vi "RelayBoard_16in16out_ZQ_TestStand.vi"(8 "On/Off":bool, 9 "Index":dbl, 10 "功能":T1(ring), 11 "ComPort":string) -> (2 "DI Status":bool, 3 "数组":bool[](array[boolean]))   [LabVIEW 2018]
uses:
  <vilib>/Instr/_visa.llb/VISA Configure Serial Port (Instr).vi
panel:
  out "数组 2":bool[](array[boolean])
  out "连接状态":bool
  in  "全部断开":bool
  in  "全部闭合":bool
  in  "OUT 16":bool
  in  "OUT 15":bool
  in  "OUT 14":bool
  in  "OUT 13":bool
  in  "OUT 12":bool
  in  "OUT 11":bool
  in  "OUT 10":bool
  in  "OUT 9":bool
  in  "OUT 8":bool
  in  "OUT 7":bool
  in  "OUT 6":bool
  in  "OUT 5":bool
  in  "OUT 4":bool
  in  "OUT 3":bool
  in  "打开端口":bool
  in  "停止":bool
  in  "OUT 2":bool
  in  "OUT 1":bool
  in  "VISA resource name":refnum<visa-resource-name> caption="VISA资源名称"
  # "智嵌IO控制板_调用"
  # "X1"
  # "X2"
  # "X3"
  # "X4"
  # "X5"
  # "X6"
  # "X7"
  # "X8"
  # "X9"
  # "X10"
  # "X11"
  # "X12"
  # "X13"
  # "X14"
  # "X15"
  # "X16"
  # "X1"
  # "X2"
  # "X3"
  # "X4"
  # "X5"
  # "X6"
  # "X7"
  # "X8"
  # "X9"
  # "X10"
  # "X11"
  # "X12"
  # "X13"
  # "X14"
  # "X15"
  # "X16"
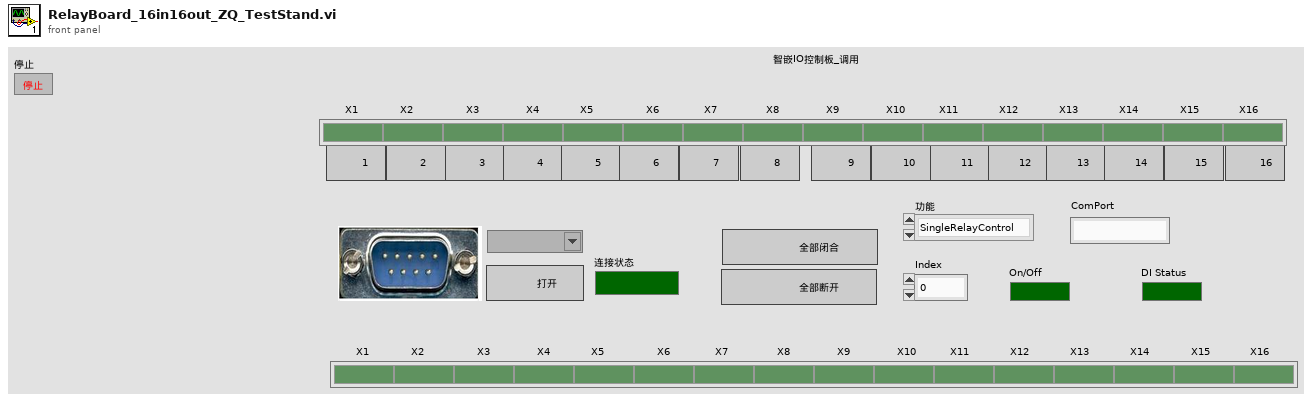
[diagram p1: front panel]
types:
  T1 = enum16{"SingleRelayControl", "AllRelaysControl", "OpenComPort", "CloseComPort", "ReadDI"}
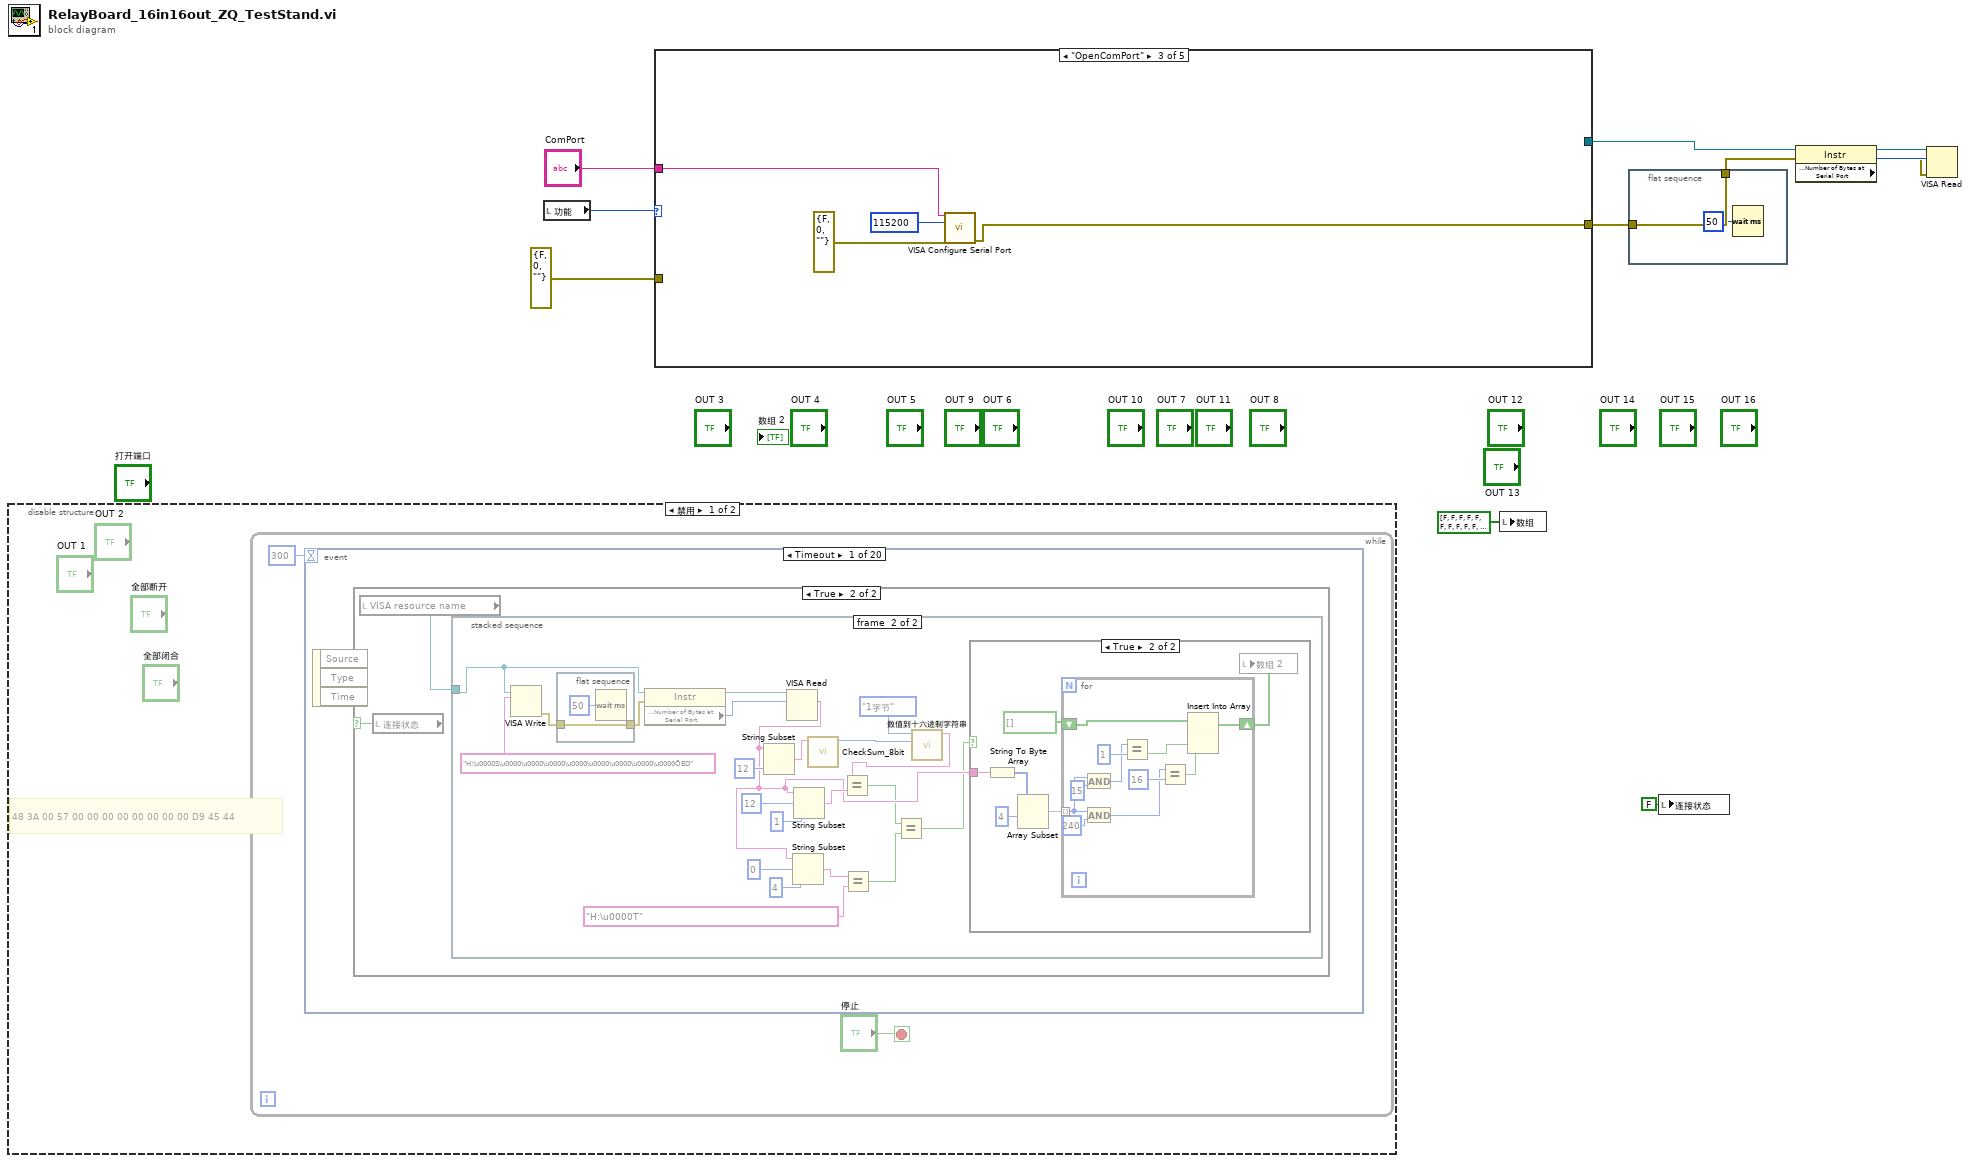
[diagram p0: block diagram]
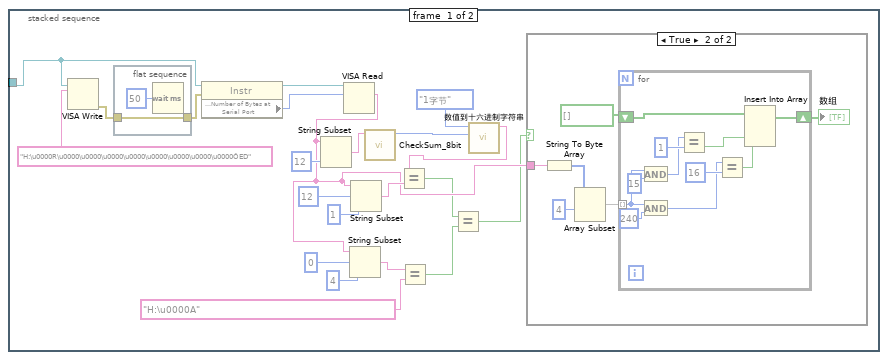
[diagram p3: hidden frame]
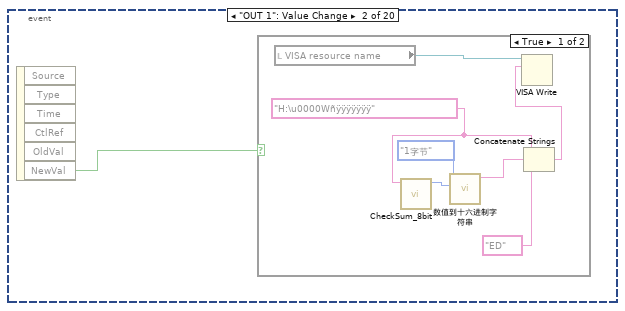
[diagram p6: hidden frame]
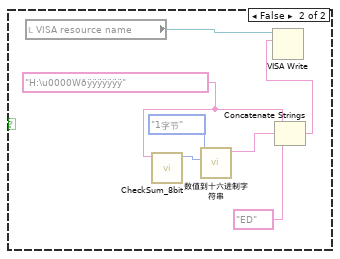
[diagram p7: hidden frame]
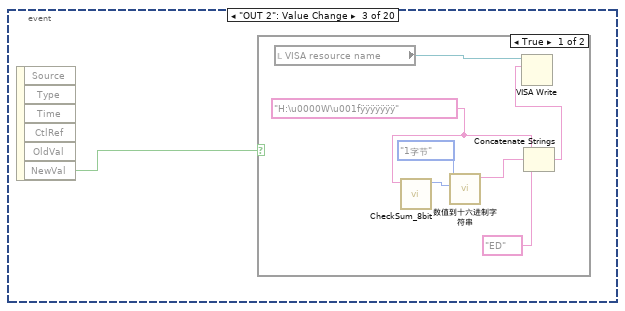
[diagram p8: hidden frame]
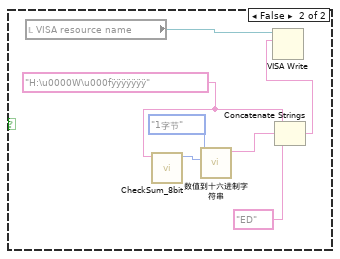
[diagram p9: hidden frame]
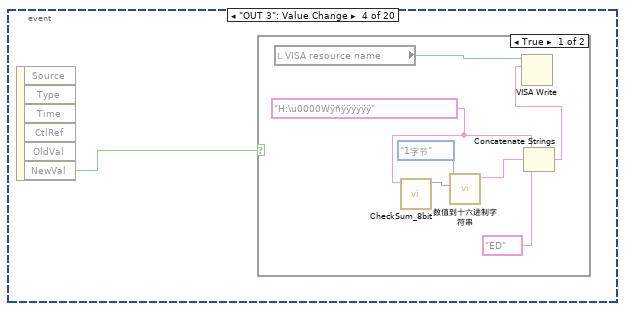
[diagram p10: hidden frame]
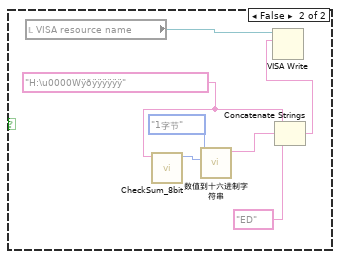
[diagram p11: hidden frame]
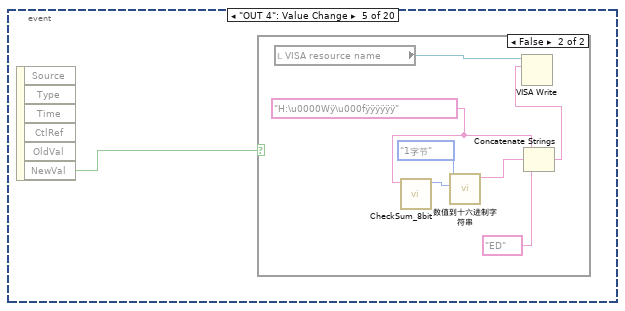
[diagram p12: hidden frame]
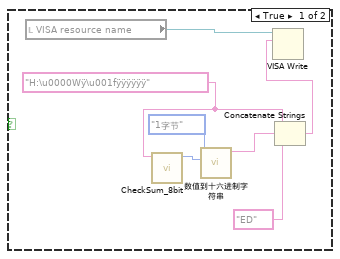
[diagram p13: hidden frame]
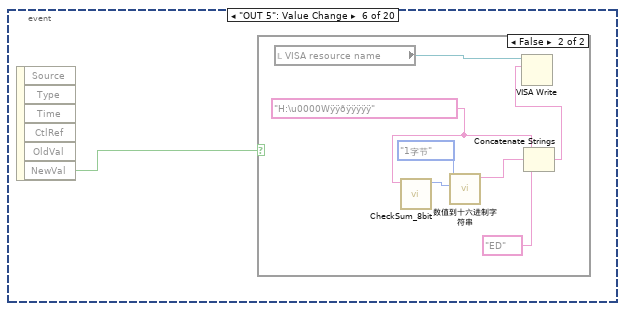
[diagram p14: hidden frame]
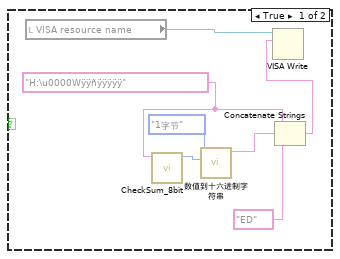
[diagram p15: hidden frame]
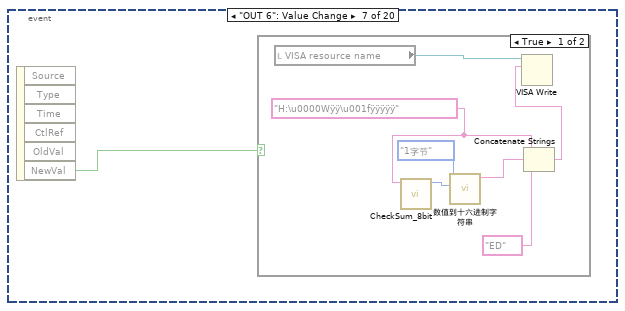
[diagram p16: hidden frame]
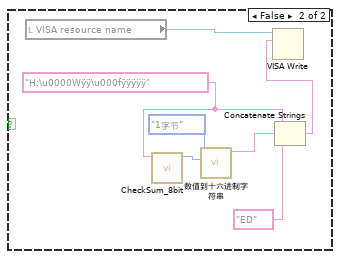
[diagram p17: hidden frame]
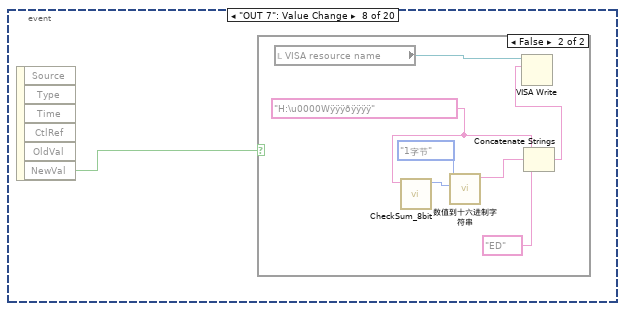
[diagram p18: hidden frame]
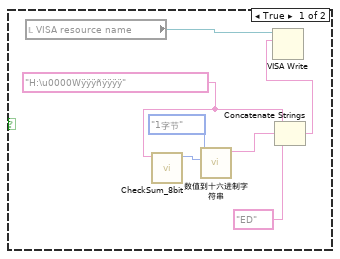
[diagram p19: hidden frame]
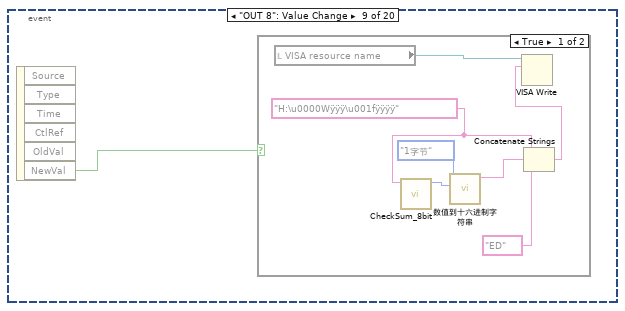
[diagram p20: hidden frame]
diagram:
  n1 = disable-structure shown="禁用" {
    frame Disabled {
      # "48 3A 00 57 00 00 00 00 00 00 00 00 D9 45 44"
      n2 = while {
        stop <- "停止" stop-if-true
        n3 = event shown="[0] Timeout" {
          selector: _ -> [_ _ _ _ _ _ _ _ _ _ _ _ _ _ _ _ _ _ _ _]
          dyn-events: _ -> [_ _ _ _ _ _ _ _ _ _ _ _ _ _ _ _ _ _ _ _]
          timeout: 300 -> [_ _ _ _ _ _ _ _ _ _ _ _ _ _ _ _ _ _ _ _]
          event Timeout {
            n4 = event-data() -> ()  [unwired: 1 in, 3 out]
            n5 = local read "连接状态"() -> (w14:bool)
            n6 = case shown="True" w14 {
              frame False {
              }
              frame True {
                n7 = local read "VISA resource name"() -> (w15:refnum<visa-resource-name>)
                n8 = stacked-sequence {
                  tunnel: w15 -> [w32 w73]
                  frame #0 {
                    n9 = VISA Write(VISA resource name=w32, write buffer="H:\u0000R\u0000\u0000\u0000\u0000\u0000\u0000\u0000\u0000ÔED" ("写入缓冲区")) -> (error out=w33:errorcluster)  [unwired: 1 in, 2 out]
                    n10 = flat-sequence {
                      tunnel: [w38] -> w34
                      tunnel: w33 -> [w38]
                      frame #0 {
                        n11 = Wait (ms)(milliseconds to wait=u32 50 ("等待时间（毫秒）")) -> ()  [unwired: 1 out]
                      }
                    }
                    n12 = property class="Instr"(reference=w32, error in=w34) -> (reference out=w37:refnum<visa-resource-name>, "Serial Settings:Number of Bytes at Serial Port"=w36:u32)  [unwired: 1 out]
                    n13 = VISA Read(VISA resource name=w37, byte count=w36) -> (read buffer=w21:string)  [unwired: 1 in, 3 out]
                    n14 = String Subset(string=w21, length (rest)=12 ("长度（剩余）")) -> (substring=w27:string)  [unwired: 1 in]
                    n15 = String Subset(string=w21, offset (0)=0 ("偏移量(0)"), length (rest)=4 ("长度（剩余）")) -> (substring=w20:string)
                    n16 = String Subset(string=w21, offset (0)=12 ("偏移量(0)"), length (rest)=1 ("长度（剩余）")) -> (substring=w28:string)
                    n17 = call "CheckSum_8bit.vi"("字符串"=w27) -> ("和"=w25:u32)  [unwired: 10 in]
                    n18 = Equal?(x=w20, y="H:\u0000A" ("写入缓冲区")) -> (x = y?=w17:bool)
                    n19 = call "数值到十六进制字符串.vi"("Numeric"=w25, "转换字节数"=enum16{"1字节", "2字节", "4字节", "3字节"}."1字节") -> ("转换结果"=w24:string)  [unwired: 8 in, 1 out]
                    n20 = Equal?(x=w24, y=w28) -> (x = y?=w18:bool)
                    n21 = Equal?(x=w18, y=w17) -> (x = y?=w16:bool)
                    n22 = case shown="True" w16 {
                      tunnel: w21 -> [_ w45]
                      frame False {
                      }
                      frame True {
                        n23 = String To Byte Array(string=w45) -> (unsigned byte array=w44:u8[])
                        n24 = Array Subset(array=w44, index=4 ("索引")) -> (w42:u8[])  [unwired: 1 in]
                        n25 = for {
                          tunnel: w42 -> [w49] mode=indexing
                          shift-right: [w51] -> w40
                          shift-left: bool[] [] -> [w54]
                          n26 = And(x=w49, y=u8 15) -> (x .and. y?=w47:u8)
                          n27 = And(x=w49, y=u8 240) -> (x .and. y?=w46:u8)
                          n28 = Equal?(x=w47, y=u8 1) -> (x = y?=w53:bool)
                          n29 = Equal?(x=w46, y=u8 16) -> (x = y?=w52:bool)
                          n30 = Insert Into Array(array=w54, new element #1=w53, new element #2=w52) -> (w51:bool[])  [unwired: 1 in]
                        }
                        "数组" <- w40
                      }
                    }
                  }
                  frame #1 {
                    n31 = VISA Write(VISA resource name=w73, write buffer="H:\u0000S\u0000\u0000\u0000\u0000\u0000\u0000\u0000\u0000ÕED" ("写入缓冲区")) -> (error out=w74:errorcluster)  [unwired: 1 in, 2 out]
                    n32 = flat-sequence {
                      tunnel: [w79] -> w75
                      tunnel: w74 -> [w79]
                      frame #0 {
                        n33 = Wait (ms)(milliseconds to wait=u32 50 ("等待时间（毫秒）")) -> ()  [unwired: 1 out]
                      }
                    }
                    n34 = property class="Instr"(reference=w73, error in=w75) -> (reference out=w78:refnum<visa-resource-name>, "Serial Settings:Number of Bytes at Serial Port"=w77:u32)  [unwired: 1 out]
                    n35 = VISA Read(VISA resource name=w78, byte count=w77) -> (read buffer=w62:string)  [unwired: 1 in, 3 out]
                    n36 = String Subset(string=w62, length (rest)=12 ("长度（剩余）")) -> (substring=w68:string)  [unwired: 1 in]
                    n37 = String Subset(string=w62, offset (0)=0 ("偏移量(0)"), length (rest)=4 ("长度（剩余）")) -> (substring=w61:string)
                    n38 = String Subset(string=w62, offset (0)=12 ("偏移量(0)"), length (rest)=1 ("长度（剩余）")) -> (substring=w69:string)
                    n39 = call "CheckSum_8bit.vi"("字符串"=w68) -> ("和"=w66:u32)  [unwired: 10 in]
                    n40 = Equal?(x=w61, y="H:\u0000T" ("写入缓冲区")) -> (x = y?=w58:bool)
                    n41 = call "数值到十六进制字符串.vi"("Numeric"=w66, "转换字节数"=enum16{"1字节", "2字节", "4字节", "3字节"}."1字节") -> ("转换结果"=w65:string)  [unwired: 8 in, 1 out]
                    n42 = Equal?(x=w65, y=w69) -> (x = y?=w59:bool)
                    n43 = Equal?(x=w59, y=w58) -> (x = y?=w57:bool)
                    n44 = case shown="True" w57 {
                      tunnel: w62 -> [_ w86]
                      frame False {
                      }
                      frame True {
                        n45 = String To Byte Array(string=w86) -> (unsigned byte array=w85:u8[])
                        n46 = Array Subset(array=w85, index=4 ("索引")) -> (w83:u8[])  [unwired: 1 in]
                        n47 = for {
                          tunnel: w83 -> [w90] mode=indexing
                          shift-right: [w92] -> w81
                          shift-left: bool[] [] -> [w95]
                          n48 = And(x=w90, y=u8 15) -> (x .and. y?=w88:u8)
                          n49 = And(x=w90, y=u8 240) -> (x .and. y?=w87:u8)
                          n50 = Equal?(x=w88, y=u8 1) -> (x = y?=w94:bool)
                          n51 = Equal?(x=w87, y=u8 16) -> (x = y?=w93:bool)
                          n52 = Insert Into Array(array=w95, new element #1=w94, new element #2=w93) -> (w92:bool[])  [unwired: 1 in]
                        }
                        n53 = local write "数组 2"(w81) -> ()
                      }
                    }
                  }
                }
              }
            }
          }
          event "OUT 1": Value Change {
            n54 = event-data() -> ("NewVal"=w98:bool)  [unwired: 1 in, 5 out]
            n55 = case shown="True" w98 {
              frame True {
                w99 = "H:\u0000Wñÿÿÿÿÿÿÿ" ("写入缓冲区")
                n56 = local read "VISA resource name"() -> (w105:refnum<visa-resource-name>)
                n57 = call "CheckSum_8bit.vi"("字符串"=w99) -> ("和"=w104:u32)  [unwired: 10 in]
                n58 = call "数值到十六进制字符串.vi"("Numeric"=w104, "转换字节数"=enum16{"1字节", "2字节", "4字节", "3字节"}."1字节") -> ("转换结果"=w102:string)  [unwired: 8 in, 1 out]
                n59 = Concatenate Strings(w99, w102, "ED" ("写入缓冲区")) -> (w100:string)
                n60 = VISA Write(VISA resource name=w105, write buffer=w100) -> ()  [unwired: 1 in, 3 out]
              }
              frame False {
                w106 = "H:\u0000Wðÿÿÿÿÿÿÿ" ("写入缓冲区")
                n61 = local read "VISA resource name"() -> (w112:refnum<visa-resource-name>)
                n62 = call "CheckSum_8bit.vi"("字符串"=w106) -> ("和"=w111:u32)  [unwired: 10 in]
                n63 = call "数值到十六进制字符串.vi"("Numeric"=w111, "转换字节数"=enum16{"1字节", "2字节", "4字节", "3字节"}."1字节") -> ("转换结果"=w109:string)  [unwired: 8 in, 1 out]
                n64 = Concatenate Strings(w106, w109, "ED" ("写入缓冲区")) -> (w107:string)
                n65 = VISA Write(VISA resource name=w112, write buffer=w107) -> ()  [unwired: 1 in, 3 out]
              }
            }
          }
          event "OUT 2": Value Change {
            n66 = event-data() -> ("NewVal"=w113:bool)  [unwired: 1 in, 5 out]
            n67 = case shown="True" w113 {
              frame True {
                w114 = "H:\u0000W\u001fÿÿÿÿÿÿÿ" ("写入缓冲区")
                n68 = local read "VISA resource name"() -> (w120:refnum<visa-resource-name>)
                n69 = call "CheckSum_8bit.vi"("字符串"=w114) -> ("和"=w119:u32)  [unwired: 10 in]
                n70 = call "数值到十六进制字符串.vi"("Numeric"=w119, "转换字节数"=enum16{"1字节", "2字节", "4字节", "3字节"}."1字节") -> ("转换结果"=w117:string)  [unwired: 8 in, 1 out]
                n71 = Concatenate Strings(w114, w117, "ED" ("写入缓冲区")) -> (w115:string)
                n72 = VISA Write(VISA resource name=w120, write buffer=w115) -> ()  [unwired: 1 in, 3 out]
              }
              frame False {
                w121 = "H:\u0000W\u000fÿÿÿÿÿÿÿ" ("写入缓冲区")
                n73 = local read "VISA resource name"() -> (w127:refnum<visa-resource-name>)
                n74 = call "CheckSum_8bit.vi"("字符串"=w121) -> ("和"=w126:u32)  [unwired: 10 in]
                n75 = call "数值到十六进制字符串.vi"("Numeric"=w126, "转换字节数"=enum16{"1字节", "2字节", "4字节", "3字节"}."1字节") -> ("转换结果"=w124:string)  [unwired: 8 in, 1 out]
                n76 = Concatenate Strings(w121, w124, "ED" ("写入缓冲区")) -> (w122:string)
                n77 = VISA Write(VISA resource name=w127, write buffer=w122) -> ()  [unwired: 1 in, 3 out]
              }
            }
          }
          event "OUT 3": Value Change {
            n78 = event-data() -> ("NewVal"=w128:bool)  [unwired: 1 in, 5 out]
            n79 = case shown="True" w128 {
              frame True {
                w129 = "H:\u0000Wÿñÿÿÿÿÿÿ" ("写入缓冲区")
                n80 = local read "VISA resource name"() -> (w135:refnum<visa-resource-name>)
                n81 = call "CheckSum_8bit.vi"("字符串"=w129) -> ("和"=w134:u32)  [unwired: 10 in]
                n82 = call "数值到十六进制字符串.vi"("Numeric"=w134, "转换字节数"=enum16{"1字节", "2字节", "4字节", "3字节"}."1字节") -> ("转换结果"=w132:string)  [unwired: 8 in, 1 out]
                n83 = Concatenate Strings(w129, w132, "ED" ("写入缓冲区")) -> (w130:string)
                n84 = VISA Write(VISA resource name=w135, write buffer=w130) -> ()  [unwired: 1 in, 3 out]
              }
              frame False {
                w136 = "H:\u0000Wÿðÿÿÿÿÿÿ" ("写入缓冲区")
                n85 = local read "VISA resource name"() -> (w142:refnum<visa-resource-name>)
                n86 = call "CheckSum_8bit.vi"("字符串"=w136) -> ("和"=w141:u32)  [unwired: 10 in]
                n87 = call "数值到十六进制字符串.vi"("Numeric"=w141, "转换字节数"=enum16{"1字节", "2字节", "4字节", "3字节"}."1字节") -> ("转换结果"=w139:string)  [unwired: 8 in, 1 out]
                n88 = Concatenate Strings(w136, w139, "ED" ("写入缓冲区")) -> (w137:string)
                n89 = VISA Write(VISA resource name=w142, write buffer=w137) -> ()  [unwired: 1 in, 3 out]
              }
            }
          }
          event "OUT 4": Value Change {
            n90 = event-data() -> ("NewVal"=w143:bool)  [unwired: 1 in, 5 out]
            n91 = case shown="False" w143 {
              frame True {
                w144 = "H:\u0000Wÿ\u001fÿÿÿÿÿÿ" ("写入缓冲区")
                n92 = local read "VISA resource name"() -> (w150:refnum<visa-resource-name>)
                n93 = call "CheckSum_8bit.vi"("字符串"=w144) -> ("和"=w149:u32)  [unwired: 10 in]
                n94 = call "数值到十六进制字符串.vi"("Numeric"=w149, "转换字节数"=enum16{"1字节", "2字节", "4字节", "3字节"}."1字节") -> ("转换结果"=w147:string)  [unwired: 8 in, 1 out]
                n95 = Concatenate Strings(w144, w147, "ED" ("写入缓冲区")) -> (w145:string)
                n96 = VISA Write(VISA resource name=w150, write buffer=w145) -> ()  [unwired: 1 in, 3 out]
              }
              frame False {
                w151 = "H:\u0000Wÿ\u000fÿÿÿÿÿÿ" ("写入缓冲区")
                n97 = local read "VISA resource name"() -> (w157:refnum<visa-resource-name>)
                n98 = call "CheckSum_8bit.vi"("字符串"=w151) -> ("和"=w156:u32)  [unwired: 10 in]
                n99 = call "数值到十六进制字符串.vi"("Numeric"=w156, "转换字节数"=enum16{"1字节", "2字节", "4字节", "3字节"}."1字节") -> ("转换结果"=w154:string)  [unwired: 8 in, 1 out]
                n100 = Concatenate Strings(w151, w154, "ED" ("写入缓冲区")) -> (w152:string)
                n101 = VISA Write(VISA resource name=w157, write buffer=w152) -> ()  [unwired: 1 in, 3 out]
              }
            }
          }
          event "OUT 5": Value Change {
            n102 = event-data() -> ("NewVal"=w158:bool)  [unwired: 1 in, 5 out]
            n103 = case shown="False" w158 {
              frame True {
                w159 = "H:\u0000Wÿÿñÿÿÿÿÿ" ("写入缓冲区")
                n104 = local read "VISA resource name"() -> (w165:refnum<visa-resource-name>)
                n105 = call "CheckSum_8bit.vi"("字符串"=w159) -> ("和"=w164:u32)  [unwired: 10 in]
                n106 = call "数值到十六进制字符串.vi"("Numeric"=w164, "转换字节数"=enum16{"1字节", "2字节", "4字节", "3字节"}."1字节") -> ("转换结果"=w162:string)  [unwired: 8 in, 1 out]
                n107 = Concatenate Strings(w159, w162, "ED" ("写入缓冲区")) -> (w160:string)
                n108 = VISA Write(VISA resource name=w165, write buffer=w160) -> ()  [unwired: 1 in, 3 out]
              }
              frame False {
                w166 = "H:\u0000Wÿÿðÿÿÿÿÿ" ("写入缓冲区")
                n109 = local read "VISA resource name"() -> (w172:refnum<visa-resource-name>)
                n110 = call "CheckSum_8bit.vi"("字符串"=w166) -> ("和"=w171:u32)  [unwired: 10 in]
                n111 = call "数值到十六进制字符串.vi"("Numeric"=w171, "转换字节数"=enum16{"1字节", "2字节", "4字节", "3字节"}."1字节") -> ("转换结果"=w169:string)  [unwired: 8 in, 1 out]
                n112 = Concatenate Strings(w166, w169, "ED" ("写入缓冲区")) -> (w167:string)
                n113 = VISA Write(VISA resource name=w172, write buffer=w167) -> ()  [unwired: 1 in, 3 out]
              }
            }
          }
          event "OUT 6": Value Change {
            n114 = event-data() -> ("NewVal"=w173:bool)  [unwired: 1 in, 5 out]
            n115 = case shown="True" w173 {
              frame True {
                w174 = "H:\u0000Wÿÿ\u001fÿÿÿÿÿ" ("写入缓冲区")
                n116 = local read "VISA resource name"() -> (w180:refnum<visa-resource-name>)
                n117 = call "CheckSum_8bit.vi"("字符串"=w174) -> ("和"=w179:u32)  [unwired: 10 in]
                n118 = call "数值到十六进制字符串.vi"("Numeric"=w179, "转换字节数"=enum16{"1字节", "2字节", "4字节", "3字节"}."1字节") -> ("转换结果"=w177:string)  [unwired: 8 in, 1 out]
                n119 = Concatenate Strings(w174, w177, "ED" ("写入缓冲区")) -> (w175:string)
                n120 = VISA Write(VISA resource name=w180, write buffer=w175) -> ()  [unwired: 1 in, 3 out]
              }
              frame False {
                w181 = "H:\u0000Wÿÿ\u000fÿÿÿÿÿ" ("写入缓冲区")
                n121 = local read "VISA resource name"() -> (w187:refnum<visa-resource-name>)
                n122 = call "CheckSum_8bit.vi"("字符串"=w181) -> ("和"=w186:u32)  [unwired: 10 in]
                n123 = call "数值到十六进制字符串.vi"("Numeric"=w186, "转换字节数"=enum16{"1字节", "2字节", "4字节", "3字节"}."1字节") -> ("转换结果"=w184:string)  [unwired: 8 in, 1 out]
                n124 = Concatenate Strings(w181, w184, "ED" ("写入缓冲区")) -> (w182:string)
                n125 = VISA Write(VISA resource name=w187, write buffer=w182) -> ()  [unwired: 1 in, 3 out]
              }
            }
          }
          event "OUT 7": Value Change {
            n126 = event-data() -> ("NewVal"=w188:bool)  [unwired: 1 in, 5 out]
            n127 = case shown="False" w188 {
              frame True {
                w189 = "H:\u0000Wÿÿÿñÿÿÿÿ" ("写入缓冲区")
                n128 = local read "VISA resource name"() -> (w195:refnum<visa-resource-name>)
                n129 = call "CheckSum_8bit.vi"("字符串"=w189) -> ("和"=w194:u32)  [unwired: 10 in]
                n130 = call "数值到十六进制字符串.vi"("Numeric"=w194, "转换字节数"=enum16{"1字节", "2字节", "4字节", "3字节"}."1字节") -> ("转换结果"=w192:string)  [unwired: 8 in, 1 out]
                n131 = Concatenate Strings(w189, w192, "ED" ("写入缓冲区")) -> (w190:string)
                n132 = VISA Write(VISA resource name=w195, write buffer=w190) -> ()  [unwired: 1 in, 3 out]
              }
              frame False {
                w196 = "H:\u0000Wÿÿÿðÿÿÿÿ" ("写入缓冲区")
                n133 = local read "VISA resource name"() -> (w202:refnum<visa-resource-name>)
                n134 = call "CheckSum_8bit.vi"("字符串"=w196) -> ("和"=w201:u32)  [unwired: 10 in]
                n135 = call "数值到十六进制字符串.vi"("Numeric"=w201, "转换字节数"=enum16{"1字节", "2字节", "4字节", "3字节"}."1字节") -> ("转换结果"=w199:string)  [unwired: 8 in, 1 out]
                n136 = Concatenate Strings(w196, w199, "ED" ("写入缓冲区")) -> (w197:string)
                n137 = VISA Write(VISA resource name=w202, write buffer=w197) -> ()  [unwired: 1 in, 3 out]
              }
            }
          }
          event "OUT 8": Value Change {
            n138 = event-data() -> ("NewVal"=w203:bool)  [unwired: 1 in, 5 out]
            n139 = case shown="True" w203 {
              frame True {
                w204 = "H:\u0000Wÿÿÿ\u001fÿÿÿÿ" ("写入缓冲区")
                n140 = local read "VISA resource name"() -> (w210:refnum<visa-resource-name>)
                n141 = call "CheckSum_8bit.vi"("字符串"=w204) -> ("和"=w209:u32)  [unwired: 10 in]
                n142 = call "数值到十六进制字符串.vi"("Numeric"=w209, "转换字节数"=enum16{"1字节", "2字节", "4字节", "3字节"}."1字节") -> ("转换结果"=w207:string)  [unwired: 8 in, 1 out]
                n143 = Concatenate Strings(w204, w207, "ED" ("写入缓冲区")) -> (w205:string)
                n144 = VISA Write(VISA resource name=w210, write buffer=w205) -> ()  [unwired: 1 in, 3 out]
              }
              frame False {
                w211 = "H:\u0000Wÿÿÿ\u000fÿÿÿÿ" ("写入缓冲区")
                n145 = local read "VISA resource name"() -> (w217:refnum<visa-resource-name>)
                n146 = call "CheckSum_8bit.vi"("字符串"=w211) -> ("和"=w216:u32)  [unwired: 10 in]
                n147 = call "数值到十六进制字符串.vi"("Numeric"=w216, "转换字节数"=enum16{"1字节", "2字节", "4字节", "3字节"}."1字节") -> ("转换结果"=w214:string)  [unwired: 8 in, 1 out]
                n148 = Concatenate Strings(w211, w214, "ED" ("写入缓冲区")) -> (w212:string)
                n149 = VISA Write(VISA resource name=w217, write buffer=w212) -> ()  [unwired: 1 in, 3 out]
              }
            }
          }
          event "OUT 9": Value Change {
            n150 = event-data() -> ("NewVal"=w218:bool)  [unwired: 1 in, 5 out]
            n151 = case shown="True" w218 {
              frame True {
                w219 = "H:\u0000Wÿÿÿÿñÿÿÿ" ("写入缓冲区")
                n152 = local read "VISA resource name"() -> (w225:refnum<visa-resource-name>)
                n153 = call "CheckSum_8bit.vi"("字符串"=w219) -> ("和"=w224:u32)  [unwired: 10 in]
                n154 = call "数值到十六进制字符串.vi"("Numeric"=w224, "转换字节数"=enum16{"1字节", "2字节", "4字节", "3字节"}."1字节") -> ("转换结果"=w222:string)  [unwired: 8 in, 1 out]
                n155 = Concatenate Strings(w219, w222, "ED" ("写入缓冲区")) -> (w220:string)
                n156 = VISA Write(VISA resource name=w225, write buffer=w220) -> ()  [unwired: 1 in, 3 out]
              }
              frame False {
                w226 = "H:\u0000Wÿÿÿÿðÿÿÿ" ("写入缓冲区")
                n157 = local read "VISA resource name"() -> (w232:refnum<visa-resource-name>)
                n158 = call "CheckSum_8bit.vi"("字符串"=w226) -> ("和"=w231:u32)  [unwired: 10 in]
                n159 = call "数值到十六进制字符串.vi"("Numeric"=w231, "转换字节数"=enum16{"1字节", "2字节", "4字节", "3字节"}."1字节") -> ("转换结果"=w229:string)  [unwired: 8 in, 1 out]
                n160 = Concatenate Strings(w226, w229, "ED" ("写入缓冲区")) -> (w227:string)
                n161 = VISA Write(VISA resource name=w232, write buffer=w227) -> ()  [unwired: 1 in, 3 out]
              }
            }
          }
          event "OUT 10": Value Change {
            n162 = event-data() -> ("NewVal"=w233:bool)  [unwired: 1 in, 5 out]
            n163 = case shown="False" w233 {
              frame True {
                w234 = "H:\u0000Wÿÿÿÿ\u001fÿÿÿ" ("写入缓冲区")
                n164 = local read "VISA resource name"() -> (w240:refnum<visa-resource-name>)
                n165 = call "CheckSum_8bit.vi"("字符串"=w234) -> ("和"=w239:u32)  [unwired: 10 in]
                n166 = call "数值到十六进制字符串.vi"("Numeric"=w239, "转换字节数"=enum16{"1字节", "2字节", "4字节", "3字节"}."1字节") -> ("转换结果"=w237:string)  [unwired: 8 in, 1 out]
                n167 = Concatenate Strings(w234, w237, "ED" ("写入缓冲区")) -> (w235:string)
                n168 = VISA Write(VISA resource name=w240, write buffer=w235) -> ()  [unwired: 1 in, 3 out]
              }
              frame False {
                w241 = "H:\u0000Wÿÿÿÿ\u000fÿÿÿ" ("写入缓冲区")
                n169 = local read "VISA resource name"() -> (w247:refnum<visa-resource-name>)
                n170 = call "CheckSum_8bit.vi"("字符串"=w241) -> ("和"=w246:u32)  [unwired: 10 in]
                n171 = call "数值到十六进制字符串.vi"("Numeric"=w246, "转换字节数"=enum16{"1字节", "2字节", "4字节", "3字节"}."1字节") -> ("转换结果"=w244:string)  [unwired: 8 in, 1 out]
                n172 = Concatenate Strings(w241, w244, "ED" ("写入缓冲区")) -> (w242:string)
                n173 = VISA Write(VISA resource name=w247, write buffer=w242) -> ()  [unwired: 1 in, 3 out]
              }
            }
          }
          event "OUT 11": Value Change {
            n174 = event-data() -> ("NewVal"=w248:bool)  [unwired: 1 in, 5 out]
            n175 = case shown="False" w248 {
              frame True {
                w249 = "H:\u0000Wÿÿÿÿÿñÿÿ" ("写入缓冲区")
                n176 = local read "VISA resource name"() -> (w255:refnum<visa-resource-name>)
                n177 = call "CheckSum_8bit.vi"("字符串"=w249) -> ("和"=w254:u32)  [unwired: 10 in]
                n178 = call "数值到十六进制字符串.vi"("Numeric"=w254, "转换字节数"=enum16{"1字节", "2字节", "4字节", "3字节"}."1字节") -> ("转换结果"=w252:string)  [unwired: 8 in, 1 out]
                n179 = Concatenate Strings(w249, w252, "ED" ("写入缓冲区")) -> (w250:string)
                n180 = VISA Write(VISA resource name=w255, write buffer=w250) -> ()  [unwired: 1 in, 3 out]
              }
              frame False {
                w256 = "H:\u0000Wÿÿÿÿÿðÿÿ" ("写入缓冲区")
                n181 = local read "VISA resource name"() -> (w262:refnum<visa-resource-name>)
                n182 = call "CheckSum_8bit.vi"("字符串"=w256) -> ("和"=w261:u32)  [unwired: 10 in]
                n183 = call "数值到十六进制字符串.vi"("Numeric"=w261, "转换字节数"=enum16{"1字节", "2字节", "4字节", "3字节"}."1字节") -> ("转换结果"=w259:string)  [unwired: 8 in, 1 out]
                n184 = Concatenate Strings(w256, w259, "ED" ("写入缓冲区")) -> (w257:string)
                n185 = VISA Write(VISA resource name=w262, write buffer=w257) -> ()  [unwired: 1 in, 3 out]
              }
            }
          }
          event "OUT 12": Value Change {
            n186 = event-data() -> ("NewVal"=w263:bool)  [unwired: 1 in, 5 out]
            n187 = case shown="True" w263 {
              frame True {
                w264 = "H:\u0000Wÿÿÿÿÿ\u001fÿÿ" ("写入缓冲区")
                n188 = local read "VISA resource name"() -> (w270:refnum<visa-resource-name>)
                n189 = call "CheckSum_8bit.vi"("字符串"=w264) -> ("和"=w269:u32)  [unwired: 10 in]
                n190 = call "数值到十六进制字符串.vi"("Numeric"=w269, "转换字节数"=enum16{"1字节", "2字节", "4字节", "3字节"}."1字节") -> ("转换结果"=w267:string)  [unwired: 8 in, 1 out]
                n191 = Concatenate Strings(w264, w267, "ED" ("写入缓冲区")) -> (w265:string)
                n192 = VISA Write(VISA resource name=w270, write buffer=w265) -> ()  [unwired: 1 in, 3 out]
              }
              frame False {
                w271 = "H:\u0000Wÿÿÿÿÿ\u000fÿÿ" ("写入缓冲区")
                n193 = local read "VISA resource name"() -> (w277:refnum<visa-resource-name>)
                n194 = call "CheckSum_8bit.vi"("字符串"=w271) -> ("和"=w276:u32)  [unwired: 10 in]
                n195 = call "数值到十六进制字符串.vi"("Numeric"=w276, "转换字节数"=enum16{"1字节", "2字节", "4字节", "3字节"}."1字节") -> ("转换结果"=w274:string)  [unwired: 8 in, 1 out]
                n196 = Concatenate Strings(w271, w274, "ED" ("写入缓冲区")) -> (w272:string)
                n197 = VISA Write(VISA resource name=w277, write buffer=w272) -> ()  [unwired: 1 in, 3 out]
              }
            }
          }
          event "OUT 13": Value Change {
            n198 = event-data() -> ("NewVal"=w278:bool)  [unwired: 1 in, 5 out]
            n199 = case shown="True" w278 {
              frame True {
                w279 = "H:\u0000Wÿÿÿÿÿÿñÿ" ("写入缓冲区")
                n200 = local read "VISA resource name"() -> (w285:refnum<visa-resource-name>)
                n201 = call "CheckSum_8bit.vi"("字符串"=w279) -> ("和"=w284:u32)  [unwired: 10 in]
                n202 = call "数值到十六进制字符串.vi"("Numeric"=w284, "转换字节数"=enum16{"1字节", "2字节", "4字节", "3字节"}."1字节") -> ("转换结果"=w282:string)  [unwired: 8 in, 1 out]
                n203 = Concatenate Strings(w279, w282, "ED" ("写入缓冲区")) -> (w280:string)
                n204 = VISA Write(VISA resource name=w285, write buffer=w280) -> ()  [unwired: 1 in, 3 out]
              }
              frame False {
                w286 = "H:\u0000Wÿÿÿÿÿÿðÿ" ("写入缓冲区")
                n205 = local read "VISA resource name"() -> (w292:refnum<visa-resource-name>)
                n206 = call "CheckSum_8bit.vi"("字符串"=w286) -> ("和"=w291:u32)  [unwired: 10 in]
                n207 = call "数值到十六进制字符串.vi"("Numeric"=w291, "转换字节数"=enum16{"1字节", "2字节", "4字节", "3字节"}."1字节") -> ("转换结果"=w289:string)  [unwired: 8 in, 1 out]
                n208 = Concatenate Strings(w286, w289, "ED" ("写入缓冲区")) -> (w287:string)
                n209 = VISA Write(VISA resource name=w292, write buffer=w287) -> ()  [unwired: 1 in, 3 out]
              }
            }
          }
          event "OUT 14": Value Change {
            n210 = event-data() -> ("NewVal"=w293:bool)  [unwired: 1 in, 5 out]
            n211 = case shown="False" w293 {
              frame True {
                w294 = "H:\u0000Wÿÿÿÿÿÿ\u001fÿ" ("写入缓冲区")
                n212 = local read "VISA resource name"() -> (w300:refnum<visa-resource-name>)
                n213 = call "CheckSum_8bit.vi"("字符串"=w294) -> ("和"=w299:u32)  [unwired: 10 in]
                n214 = call "数值到十六进制字符串.vi"("Numeric"=w299, "转换字节数"=enum16{"1字节", "2字节", "4字节", "3字节"}."1字节") -> ("转换结果"=w297:string)  [unwired: 8 in, 1 out]
                n215 = Concatenate Strings(w294, w297, "ED" ("写入缓冲区")) -> (w295:string)
                n216 = VISA Write(VISA resource name=w300, write buffer=w295) -> ()  [unwired: 1 in, 3 out]
              }
              frame False {
                w301 = "H:\u0000Wÿÿÿÿÿÿ\u000fÿ" ("写入缓冲区")
                n217 = local read "VISA resource name"() -> (w307:refnum<visa-resource-name>)
                n218 = call "CheckSum_8bit.vi"("字符串"=w301) -> ("和"=w306:u32)  [unwired: 10 in]
                n219 = call "数值到十六进制字符串.vi"("Numeric"=w306, "转换字节数"=enum16{"1字节", "2字节", "4字节", "3字节"}."1字节") -> ("转换结果"=w304:string)  [unwired: 8 in, 1 out]
                n220 = Concatenate Strings(w301, w304, "ED" ("写入缓冲区")) -> (w302:string)
                n221 = VISA Write(VISA resource name=w307, write buffer=w302) -> ()  [unwired: 1 in, 3 out]
              }
            }
          }
          event "OUT 15": Value Change {
            n222 = event-data() -> ("NewVal"=w308:bool)  [unwired: 1 in, 5 out]
            n223 = case shown="True" w308 {
              frame True {
                w309 = "H:\u0000Wÿÿÿÿÿÿÿñ" ("写入缓冲区")
                n224 = local read "VISA resource name"() -> (w315:refnum<visa-resource-name>)
                n225 = call "CheckSum_8bit.vi"("字符串"=w309) -> ("和"=w314:u32)  [unwired: 10 in]
                n226 = call "数值到十六进制字符串.vi"("Numeric"=w314, "转换字节数"=enum16{"1字节", "2字节", "4字节", "3字节"}."1字节") -> ("转换结果"=w312:string)  [unwired: 8 in, 1 out]
                n227 = Concatenate Strings(w309, w312, "ED" ("写入缓冲区")) -> (w310:string)
                n228 = VISA Write(VISA resource name=w315, write buffer=w310) -> ()  [unwired: 1 in, 3 out]
              }
              frame False {
                w316 = "H:\u0000Wÿÿÿÿÿÿÿð" ("写入缓冲区")
                n229 = local read "VISA resource name"() -> (w322:refnum<visa-resource-name>)
                n230 = call "CheckSum_8bit.vi"("字符串"=w316) -> ("和"=w321:u32)  [unwired: 10 in]
                n231 = call "数值到十六进制字符串.vi"("Numeric"=w321, "转换字节数"=enum16{"1字节", "2字节", "4字节", "3字节"}."1字节") -> ("转换结果"=w319:string)  [unwired: 8 in, 1 out]
                n232 = Concatenate Strings(w316, w319, "ED" ("写入缓冲区")) -> (w317:string)
                n233 = VISA Write(VISA resource name=w322, write buffer=w317) -> ()  [unwired: 1 in, 3 out]
              }
            }
          }
          event "OUT 16": Value Change {
            n234 = event-data() -> ("NewVal"=w323:bool)  [unwired: 1 in, 5 out]
            n235 = case shown="False" w323 {
              frame True {
                w324 = "H:\u0000Wÿÿÿÿÿÿÿ\u001f" ("写入缓冲区")
                n236 = local read "VISA resource name"() -> (w330:refnum<visa-resource-name>)
                n237 = call "CheckSum_8bit.vi"("字符串"=w324) -> ("和"=w329:u32)  [unwired: 10 in]
                n238 = call "数值到十六进制字符串.vi"("Numeric"=w329, "转换字节数"=enum16{"1字节", "2字节", "4字节", "3字节"}."1字节") -> ("转换结果"=w327:string)  [unwired: 8 in, 1 out]
                n239 = Concatenate Strings(w324, w327, "ED" ("写入缓冲区")) -> (w325:string)
                n240 = VISA Write(VISA resource name=w330, write buffer=w325) -> ()  [unwired: 1 in, 3 out]
              }
              frame False {
                w331 = "H:\u0000Wÿÿÿÿÿÿÿ\u000f" ("写入缓冲区")
                n241 = local read "VISA resource name"() -> (w337:refnum<visa-resource-name>)
                n242 = call "CheckSum_8bit.vi"("字符串"=w331) -> ("和"=w336:u32)  [unwired: 10 in]
                n243 = call "数值到十六进制字符串.vi"("Numeric"=w336, "转换字节数"=enum16{"1字节", "2字节", "4字节", "3字节"}."1字节") -> ("转换结果"=w334:string)  [unwired: 8 in, 1 out]
                n244 = Concatenate Strings(w331, w334, "ED" ("写入缓冲区")) -> (w332:string)
                n245 = VISA Write(VISA resource name=w337, write buffer=w332) -> ()  [unwired: 1 in, 3 out]
              }
            }
          }
          event "全部闭合": Value Change {
            w338 = "H:\u0000W\u0011\u0011\u0011\u0011\u0011\u0011\u0011\u0011" ("写入缓冲区")
            n246 = event-data() -> ()  [unwired: 1 in, 6 out]
            n247 = call "CheckSum_8bit.vi"("字符串"=w338) -> ("和"=w343:u32)  [unwired: 10 in]
            n248 = call "数值到十六进制字符串.vi"("Numeric"=w343, "转换字节数"=enum16{"1字节", "2字节", "4字节", "3字节"}."1字节") -> ("转换结果"=w341:string)  [unwired: 8 in, 1 out]
            n249 = local read "VISA resource name"() -> (w344:refnum<visa-resource-name>)
            n250 = Concatenate Strings(w338, w341, "ED" ("写入缓冲区")) -> (w339:string)
            n251 = VISA Write(VISA resource name=w344, write buffer=w339) -> ()  [unwired: 1 in, 3 out]
          }
          event "全部断开": Value Change {
            w350 = "H:\u0000W\u0000\u0000\u0000\u0000\u0000\u0000\u0000\u0000" ("写入缓冲区")
            n252 = event-data() -> ()  [unwired: 1 in, 6 out]
            n253 = invoke on="OUT 9" class="Bool" method="Reinit To Default"() -> (error out=w346:errorcluster)  [unwired: 3 in, 2 out]
            n254 = invoke on="OUT 1" class="Bool" method="Reinit To Default"() -> ()  [unwired: 3 in, 3 out]
            n255 = invoke on="OUT 2" class="Bool" method="Reinit To Default"() -> (error out=w349:errorcluster)  [unwired: 3 in, 2 out]
            n256 = invoke on="OUT 10" class="Bool" method="Reinit To Default"(error in=w346) -> ()  [unwired: 2 in, 3 out]
            n257 = invoke on="OUT 3" class="Bool" method="Reinit To Default"(error in=w349) -> (error out=w348:errorcluster)  [unwired: 2 in, 2 out]
            n258 = invoke on="OUT 11" class="Bool" method="Reinit To Default"() -> ()  [unwired: 3 in, 3 out]
            n259 = call "CheckSum_8bit.vi"("字符串"=w350) -> ("和"=w355:u32)  [unwired: 10 in]
            n260 = invoke on="OUT 4" class="Bool" method="Reinit To Default"(error in=w348) -> ()  [unwired: 2 in, 3 out]
            n261 = invoke on="OUT 12" class="Bool" method="Reinit To Default"() -> (error out=w345:errorcluster)  [unwired: 3 in, 2 out]
            n262 = local read "VISA resource name"() -> (w356:refnum<visa-resource-name>)
            n263 = call "数值到十六进制字符串.vi"("Numeric"=w355, "转换字节数"=enum16{"1字节", "2字节", "4字节", "3字节"}."1字节") -> ("转换结果"=w353:string)  [unwired: 8 in, 1 out]
            n264 = Concatenate Strings(w350, w353, "ED" ("写入缓冲区")) -> (w351:string)
            n265 = invoke on="OUT 5" class="Bool" method="Reinit To Default"() -> ()  [unwired: 3 in, 3 out]
            n266 = invoke on="OUT 13" class="Bool" method="Reinit To Default"(error in=w345) -> ()  [unwired: 2 in, 3 out]
            n267 = VISA Write(VISA resource name=w356, write buffer=w351) -> ()  [unwired: 1 in, 3 out]
            n268 = invoke on="OUT 6" class="Bool" method="Reinit To Default"() -> ()  [unwired: 3 in, 3 out]
            n269 = invoke on="OUT 14" class="Bool" method="Reinit To Default"() -> ()  [unwired: 3 in, 3 out]
            n270 = invoke on="OUT 7" class="Bool" method="Reinit To Default"() -> (error out=w347:errorcluster)  [unwired: 3 in, 2 out]
            n271 = invoke on="OUT 15" class="Bool" method="Reinit To Default"() -> ()  [unwired: 3 in, 3 out]
            n272 = invoke on="OUT 8" class="Bool" method="Reinit To Default"(error in=w347) -> ()  [unwired: 2 in, 3 out]
            n273 = invoke on="OUT 16" class="Bool" method="Reinit To Default"() -> ()  [unwired: 3 in, 3 out]
          }
          event "打开端口": Value Change {
            n274 = event-data() -> ("NewVal"=w359:bool)  [unwired: 1 in, 5 out]
            n275 = case shown="False" w359 {
              tunnel: "VISA resource name" -> [w361 w366]
              tunnel: [w360 FALSE] -> w357
              frame True {
                n276 = call-poly "VISA Configure Serial Port"("VISA resource name"=w361, "baud rate (9600)"=u32 115200) -> ("error out"=w363:errorcluster)  [unwired: 12 in, 1 out]
                n277 = Unbundle(w363) -> ("status"=w362:bool)  [unwired: 2 out]
                n278 = Not(x=w362) -> (.not. x?=w360:bool)
              }
              frame False {
                n279 = VISA Close(VISA resource name=w366) -> ()  [unwired: 1 in, 1 out]
              }
            }
            "连接状态" <- w357
          }
        }
      }
    }
    frame Enabled {
    }
  }
  n280 = local read "功能"() -> (w10:T1)
  n281 = case shown="\"OpenComPort\"" w10 {
    tunnel: "ComPort" -> [w372 w400 w422 w426 w427]
    tunnel: errorcluster {"status"=FALSE, "code"=0, "source"=""} ("错误输入（无错误）") -> [w370 _ _ w425 _]
    tunnel: [w371 w398 w420 w424 _] -> w1
    tunnel: [w367 w399 _ _ _] -> w4
    frame "SingleRelayControl", Default {
      n282 = local read "Index"() -> (w369:dbl)
      n283 = Decrement(x=w369) -> (x-1=w368:dbl)
      n284 = local read "On/Off"() -> (w373:bool)
      n285 = Index Array(array=string[] ["H:\u0000Wñÿÿÿÿÿÿÿ", "H:\u0000W\u001fÿÿÿÿÿÿÿ", "H:\u0000Wÿñÿÿÿÿÿÿ", "H:\u0000Wÿ\u001fÿÿÿÿÿÿ", "H:\u0000Wÿÿñÿÿÿÿÿ", "H:\u0000Wÿÿ\u001fÿÿÿÿÿ", "H:\u0000Wÿÿÿñÿÿÿÿ", "H:\u0000Wÿÿÿ\u001fÿÿÿÿ", "H:\u0000Wÿÿÿÿñÿÿÿ", "H:\u0000Wñÿÿÿ\u001fÿÿÿ", "H:\u0000Wñÿÿÿÿñÿÿ", "H:\u0000Wÿÿÿÿÿ\u001fÿÿ", "H:\u0000Wÿÿÿÿÿÿñÿ", "H:\u0000Wÿÿÿÿÿÿ\u001fÿ", "H:\u0000Wÿÿÿÿÿÿÿñ", "H:\u0000Wÿÿÿÿÿÿÿ\u001f"], index=w368) -> (element=w374:string)
      n286 = Index Array(array=string[] ["H:\u0000Wðÿÿÿÿÿÿÿ", "H:\u0000W\u000fÿÿÿÿÿÿÿ", "H:\u0000Wÿðÿÿÿÿÿÿ", "H:\u0000Wÿ\u000fÿÿÿÿÿÿ", "H:\u0000Wÿÿðÿÿÿÿÿ", "H:\u0000Wÿÿ\u000fÿÿÿÿÿ", "H:\u0000Wÿÿÿðÿÿÿÿ", "H:\u0000Wÿÿÿ\u000fÿÿÿÿ", "H:\u0000Wÿÿÿÿðÿÿÿ", "H:\u0000Wñÿÿÿ\u000fÿÿÿ", "H:\u0000Wñÿÿÿÿðÿÿ", "H:\u0000Wÿÿÿÿÿ\u000fÿÿ", "H:\u0000Wÿÿÿÿÿÿðÿ", "H:\u0000Wÿÿÿÿÿÿ\u000fÿ", "H:\u0000Wÿÿÿÿÿÿÿð", "H:\u0000Wÿÿÿÿÿÿÿ\u000f"], index=w368) -> (element=w375:string)
      n287 = case shown="False" w373 {
        tunnel: w372 -> [w382 w392]
        tunnel: w375 -> [_ w390]
        tunnel: w374 -> [w381 _]
        tunnel: [w380 w391] -> w371
        tunnel: w370 -> [w379 w389]
        tunnel: [w378 w388] -> w367
        frame True {
          n288 = call "CheckSum_8bit.vi"("字符串"=w381) -> ("和"=w387:u32)  [unwired: 10 in]
          n289 = call "数值到十六进制字符串.vi"("Numeric"=w387, "转换字节数"=enum16{"1字节", "2字节", "4字节", "3字节"}."1字节") -> ("转换结果"=w385:string)  [unwired: 8 in, 1 out]
          n290 = Concatenate Strings(w381, w385, "ED" ("写入缓冲区")) -> (w383:string)
          n291 = VISA Write(VISA resource name=w382, write buffer=w383, error in (no error)=w379) -> (VISA resource name out=w378:refnum<visa-resource-name>, error out=w380:errorcluster)  [unwired: 1 out]
        }
        frame False {
          n292 = call "CheckSum_8bit.vi"("字符串"=w390) -> ("和"=w397:u32)  [unwired: 10 in]
          n293 = call "数值到十六进制字符串.vi"("Numeric"=w397, "转换字节数"=enum16{"1字节", "2字节", "4字节", "3字节"}."1字节") -> ("转换结果"=w395:string)  [unwired: 8 in, 1 out]
          n294 = Concatenate Strings(w390, w395, "ED" ("写入缓冲区")) -> (w393:string)
          n295 = VISA Write(VISA resource name=w392, write buffer=w393, error in (no error)=w389) -> (VISA resource name out=w388:refnum<visa-resource-name>, error out=w391:errorcluster)  [unwired: 1 out]
        }
      }
    }
    frame "AllRelaysControl" {
      n296 = local read "On/Off"() -> (w401:bool)
      n297 = case shown="True" w401 {
        tunnel: w400 -> [w404 w413]
        tunnel: [w403 w412] -> w399
        tunnel: [w402 w411] -> w398
        frame False {
          w410 = "H:\u0000W\u0000\u0000\u0000\u0000\u0000\u0000\u0000\u0000" ("写入缓冲区")
          n298 = call "CheckSum_8bit.vi"("字符串"=w410) -> ("和"=w405:u32)  [unwired: 10 in]
          n299 = call "数值到十六进制字符串.vi"("Numeric"=w405, "转换字节数"=enum16{"1字节", "2字节", "4字节", "3字节"}."1字节") -> ("转换结果"=w407:string)  [unwired: 8 in, 1 out]
          n300 = Concatenate Strings(w410, w407, "ED" ("写入缓冲区")) -> (w409:string)
          n301 = VISA Write(VISA resource name=w404, write buffer=w409) -> (VISA resource name out=w403:refnum<visa-resource-name>, error out=w402:errorcluster)  [unwired: 1 in, 1 out]
        }
        frame True {
          w419 = "H:\u0000W\u0011\u0011\u0011\u0011\u0011\u0011\u0011\u0011" ("写入缓冲区")
          n302 = call "CheckSum_8bit.vi"("字符串"=w419) -> ("和"=w414:u32)  [unwired: 10 in]
          n303 = call "数值到十六进制字符串.vi"("Numeric"=w414, "转换字节数"=enum16{"1字节", "2字节", "4字节", "3字节"}."1字节") -> ("转换结果"=w416:string)  [unwired: 8 in, 1 out]
          n304 = Concatenate Strings(w419, w416, "ED" ("写入缓冲区")) -> (w418:string)
          n305 = VISA Write(VISA resource name=w413, write buffer=w418) -> (VISA resource name out=w412:refnum<visa-resource-name>, error out=w411:errorcluster)  [unwired: 1 in, 1 out]
        }
      }
    }
    frame "OpenComPort" {
      n306 = call-poly "VISA Configure Serial Port"("VISA resource name"=w422, "baud rate (9600)"=u32 115200, "error in (no error)"=errorcluster {"status"=FALSE, "code"=0, "source"=""}) -> ("error out"=w420:errorcluster)  [unwired: 11 in, 1 out]
    }
    frame "CloseComPort" {
      n307 = VISA Close(VISA resource name=w426, error in (no error)=w425) -> (error out=w424:errorcluster)
    }
    frame "ReadDI" {
      n308 = VISA Write(VISA resource name=w427, write buffer="H:\u0000R\u0000\u0000\u0000\u0000\u0000\u0000\u0000\u0000ÔED" ("写入缓冲区")) -> (VISA resource name out=w428:refnum<visa-resource-name>, error out=w433:errorcluster)  [unwired: 1 in, 1 out]
      n309 = flat-sequence {
        tunnel: [w450] -> w432
        tunnel: w433 -> [w450]
        frame #0 {
          n310 = Wait (ms)(milliseconds to wait=u32 100 ("等待时间（毫秒）")) -> ()  [unwired: 1 out]
        }
      }
      n311 = property class="Instr"(reference=w428, error in=w432) -> (reference out=w429:refnum<visa-resource-name>, "Serial Settings:Number of Bytes at Serial Port"=w430:u32)  [unwired: 1 out]
      n312 = VISA Read(VISA resource name=w429, byte count=w430) -> (read buffer=w444:string)  [unwired: 1 in, 3 out]
      n313 = String Subset(string=w444, length (rest)=12 ("长度（剩余）")) -> (substring=w438:string)  [unwired: 1 in]
      n314 = String Subset(string=w444, offset (0)=0 ("偏移量(0)"), length (rest)=4 ("长度（剩余）")) -> (substring=w445:string)
      n315 = String Subset(string=w444, offset (0)=12 ("偏移量(0)"), length (rest)=1 ("长度（剩余）")) -> (substring=w437:string)
      n316 = call "CheckSum_8bit.vi"("字符串"=w438) -> ("和"=w440:u32)  [unwired: 10 in]
      n317 = Equal?(x=w445, y="H:\u0000A" ("写入缓冲区")) -> (x = y?=w448:bool)
      n318 = call "数值到十六进制字符串.vi"("Numeric"=w440, "转换字节数"=enum16{"1字节", "2字节", "4字节", "3字节"}."1字节") -> ("转换结果"=w441:string)  [unwired: 8 in, 1 out]
      n319 = Equal?(x=w441, y=w437) -> (x = y?=w447:bool)
      n320 = Equal?(x=w447, y=w448) -> (x = y?=w449:bool)
      n321 = case shown="True" w449 {
        tunnel: w444 -> [_ w460]
        frame False {
        }
        frame True {
          n322 = String To Byte Array(string=w460) -> (unsigned byte array=w459:u8[])
          n323 = Array Subset(array=w459, index=4 ("索引")) -> (w457:u8[])  [unwired: 1 in]
          n324 = for {
            tunnel: w457 -> [w464] mode=indexing
            shift-right: [w466] -> w455
            shift-left: bool[] [] -> [w469]
            n325 = And(x=w464, y=u8 15) -> (x .and. y?=w462:u8)
            n326 = And(x=w464, y=u8 240) -> (x .and. y?=w461:u8)
            n327 = Equal?(x=w462, y=u8 1) -> (x = y?=w468:bool)
            n328 = Equal?(x=w461, y=u8 16) -> (x = y?=w467:bool)
            n329 = Insert Into Array(array=w469, new element #1=w468, new element #2=w467) -> (w466:bool[])  [unwired: 1 in]
          }
          n330 = local read "Index"() -> (w454:dbl)
          n331 = Decrement(x=w454) -> (x-1=w453:dbl)
          n332 = local write "数组"(w455) -> ()
          n333 = Index Array(array=w455, index=w453) -> (element=w452:bool)
          n334 = local write "DI Status"(w452) -> ()
        }
      }
    }
  }
  n335 = local write "数组"(bool[] [FALSE, FALSE, FALSE, FALSE, FALSE, FALSE, FALSE, FALSE, FALSE, FALSE, FALSE, FALSE, FALSE, FALSE, FALSE, FALSE] ("数组")) -> ()
  n336 = flat-sequence {
    tunnel: [w473] -> w2
    tunnel: w1 -> [w473]
    frame #0 {
      n337 = Wait (ms)(milliseconds to wait=u32 50 ("等待时间（毫秒）")) -> ()  [unwired: 1 out]
    }
  }
  n338 = local write "连接状态"(FALSE ("status")) -> ()
  n339 = property class="Instr"(reference=w4, error in=w2) -> (reference out=w6:refnum<visa-resource-name>, error out=w3:errorcluster, "Serial Settings:Number of Bytes at Serial Port"=w5:u32)
  n340 = VISA Read(VISA resource name=w6, byte count=w5, error in (no error)=w3) -> ()  [unwired: 4 out]
